vi "orbits_seed_laser_controller.vi"() -> ()   [LabVIEW 2014]
uses:
  <vilib>/Instr/_visa.llb/VISA Configure Serial Port (Instr).vi
panel:
  out "Temp (C)":dbl=35.4
  in  "DISABLE":bool
  in  "ENABLE":bool
  in  "Read":bool
  out "Power (mW)":dbl
  out "Temp (C)":dbl(slide)=35.4 scale=0.0..50.0
  in  "Ethernal COM Port":refnum<visa-resource-name>="COM4"
  in  "Controller Stop":bool
  in  "Control Rate (ms)":u32=1000
  out "Hardware Enabled":bool=TRUE
  out "Software Enabled":bool=TRUE
  out "Temp Stable":bool=TRUE
  in  "Which Temp?":enum16{"ETH", "PUMP", "PCB", "AMP", "CASE"}(ring)
  out "TEC Setpoint":dbl=35.52 format="%#_13g"
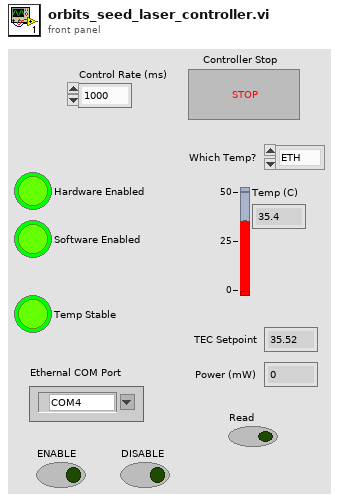
[diagram p1: front panel]
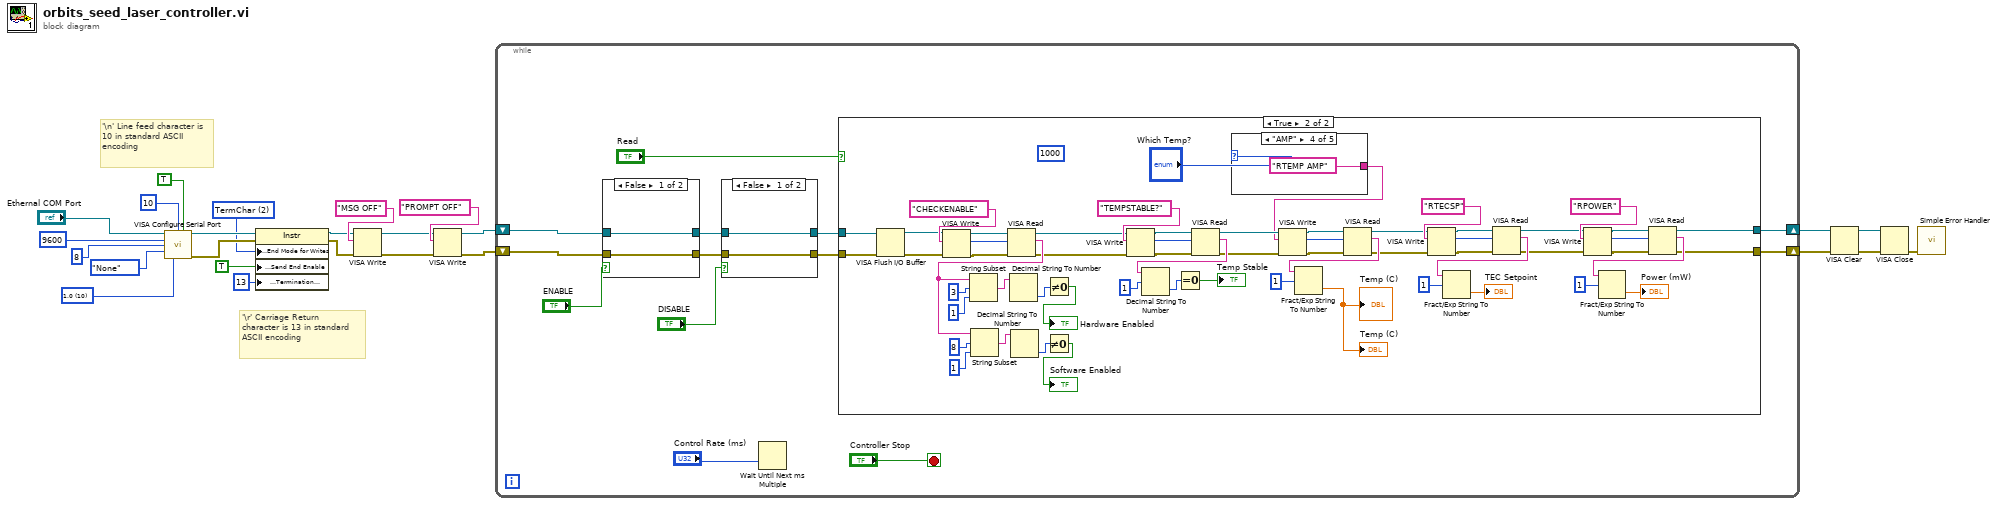
[diagram p0: block diagram]
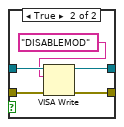
[diagram p2: hidden frame]
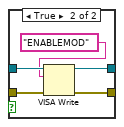
[diagram p3: hidden frame]
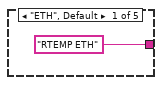
[diagram p5: hidden frame]
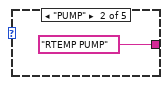
[diagram p6: hidden frame]
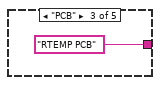
[diagram p7: hidden frame]
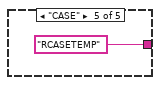
[diagram p8: hidden frame]
diagram:
  w7 = u16 10 items=["1.0"=10, "1.5"=15, "2.0"=20] ("stop bits (10: 1 bit)")
  w21 = u16 2 items=["None", "LastBit", "TermChar", "Break"] ("Serial Settings:Serial End Mode for Writes")
  # "'\\r' Carriage Return character is 13 in standard ASCII encoding"
  # "'\\n' Line feed character is 10 in standard ASCII encoding"
  n1 = call-poly "VISA Configure Serial Port"("VISA resource name"="Ethernal COM Port", "termination char\n(0xA = '\\n' = LF)"=u8 10, "Enable Termination\nChar (T)"=TRUE, "baud rate (9600)"=u32 9600, "data bits (8)"=u16 8, "parity (0:none)"=enum16{"None", "Odd", "Even", "Mark", "Space"}."None", "stop bits (10: 1 bit)"=w7) -> ("VISA resource name out"=w23:refnum<visa-resource-name>, "error out"=w24:errorcluster)  [unwired: 3 in, 4 out]
  n2 = property class="Instr"(reference=w23, error in=w24, "Serial Settings:End Mode for Writes"=w21, "Message Based Settings:Send End Enable"=TRUE, "Message Based Settings:Termination Character"=13) -> (reference out=w12:refnum<visa-resource-name>, error out=w13:errorcluster)
  n3 = VISA Write(VISA resource name=w12, write buffer="MSG OFF" ("Enable 2"), error in (no error)=w13) -> (VISA resource name out=w10:refnum<visa-resource-name>, error out=w9:errorcluster)  [unwired: 1 out]
  n4 = VISA Write(VISA resource name=w10, write buffer="PROMPT OFF" ("Enable 2"), error in (no error)=w9) -> (VISA resource name out=w6:refnum<visa-resource-name>, error out=w5:errorcluster)  [unwired: 1 out]
  n5 = while {
    shift-right: [w35] -> w3
    shift-left: w5 -> [w28]
    shift-right: [w36] -> w4
    shift-left: w6 -> [w29]
    stop <- "Controller Stop" stop-if-true
    n6 = case shown="False" "ENABLE" {
      tunnel: w29 -> [w47 w52]
      tunnel: w28 -> [w46 w51]
      tunnel: [w47 w50] -> w30
      tunnel: [w46 w49] -> w31
      frame False {
      }
      frame True {
        n7 = VISA Write(VISA resource name=w52, write buffer="ENABLEMOD" ("Enable 2"), error in (no error)=w51) -> (VISA resource name out=w50:refnum<visa-resource-name>, error out=w49:errorcluster)  [unwired: 1 out]
      }
    }
    n8 = case shown="False" "DISABLE" {
      tunnel: w30 -> [w40 w45]
      tunnel: w31 -> [w39 w44]
      tunnel: [w40 w43] -> w27
      tunnel: [w39 w42] -> w26
      frame False {
      }
      frame True {
        n9 = VISA Write(VISA resource name=w45, write buffer="DISABLEMOD" ("Enable 2"), error in (no error)=w44) -> (VISA resource name out=w43:refnum<visa-resource-name>, error out=w42:errorcluster)  [unwired: 1 out]
      }
    }
    n10 = Wait Until Next ms Multiple(millisecond multiple="Control Rate (ms)") -> ()  [unwired: 1 out]
    n11 = case shown="True" "Read" {
      tunnel: [w54 w60] -> w36
      tunnel: [w53 w59] -> w35
      tunnel: w27 -> [w54 w58]
      tunnel: w26 -> [w53 w56]
      frame False {
      }
      frame True {
        (unwired) u32 1000 ("Read Count 3")
        n12 = VISA Flush I/O Buffer(VISA resource name=w58, error in (no error)=w56) -> (VISA resource name out=w57:refnum<visa-resource-name>, error out=w55:errorcluster)  [unwired: 1 in]
        n13 = VISA Write(VISA resource name=w57, write buffer="CHECKENABLE" ("Enable 2"), error in (no error)=w55) -> (VISA resource name out=w112:refnum<visa-resource-name>, return count=w65:u32, error out=w111:errorcluster)
        n14 = VISA Read(VISA resource name=w112, byte count=w65, error in (no error)=w111) -> (VISA resource name out=w95:refnum<visa-resource-name>, read buffer=w106:string, error out=w94:errorcluster)  [unwired: 1 out]
        n15 = String Subset(string=w106, offset (0)=3, length (rest)=1) -> (substring=w105:string)
        n16 = String Subset(string=w106, offset (0)=8, length (rest)=1) -> (substring=w104:string)
        n17 = Decimal String To Number(string=w105) -> (number=w103:i32)  [unwired: 2 in, 1 out]
        n18 = Decimal String To Number(string=w104) -> (number=w100:i32)  [unwired: 2 in, 1 out]
        n19 = Not Equal To 0?(x=w100) -> (x != 0?=→"Software Enabled":bool)
        n20 = Not Equal To 0?(x=w103) -> (x != 0?=→"Hardware Enabled":bool)
        n21 = VISA Write(VISA resource name=w95, write buffer="TEMPSTABLE?" ("Enable 2"), error in (no error)=w94) -> (VISA resource name out=w98:refnum<visa-resource-name>, return count=w64:u32, error out=w97:errorcluster)
        n22 = VISA Read(VISA resource name=w98, byte count=w64, error in (no error)=w97) -> (VISA resource name out=w88:refnum<visa-resource-name>, read buffer=w96:string, error out=w87:errorcluster)  [unwired: 1 out]
        n23 = Decimal String To Number(string=w96, offset=1) -> (number=w92:i32)  [unwired: 1 in, 1 out]
        n24 = Equal To 0?(x=w92) -> (x = 0?=→"Temp Stable":bool)
        n25 = case shown="\"AMP\"" "Which Temp?" {
          tunnel: ["RTEMP ETH" ("Enable 2") "RTEMP PUMP" ("Enable 2") "RTEMP PCB" ("Enable 2") "RTEMP AMP" ("Enable 2") "RCASETEMP" ("Enable 2")] -> w86
          frame "ETH", Default {
          }
          frame "PUMP" {
          }
          frame "PCB" {
          }
          frame "AMP" {
          }
          frame "CASE" {
          }
        }
        n26 = VISA Write(VISA resource name=w88, write buffer=w86, error in (no error)=w87) -> (VISA resource name out=w90:refnum<visa-resource-name>, return count=w61:u32, error out=w89:errorcluster)
        n27 = VISA Read(VISA resource name=w90, byte count=w61, error in (no error)=w89) -> (VISA resource name out=w70:refnum<visa-resource-name>, read buffer=w85:string, error out=w69:errorcluster)  [unwired: 1 out]
        n28 = Fract/Exp String To Number(string=w85, offset=1) -> (number=→"Temp (C)" →"Temp (C)":dbl)  [unwired: 2 in, 1 out]
        n29 = VISA Write(VISA resource name=w70, write buffer="RTECSP" ("Enable 2"), error in (no error)=w69) -> (VISA resource name out=w75:refnum<visa-resource-name>, return count=w62:u32, error out=w74:errorcluster)
        n30 = VISA Read(VISA resource name=w75, byte count=w62, error in (no error)=w74) -> (VISA resource name out=w68:refnum<visa-resource-name>, read buffer=w71:string, error out=w67:errorcluster)  [unwired: 1 out]
        n31 = Fract/Exp String To Number(string=w71, offset=1) -> (number=→"TEC Setpoint":dbl)  [unwired: 2 in, 1 out]
        n32 = VISA Write(VISA resource name=w68, write buffer="RPOWER" ("Enable 2"), error in (no error)=w67) -> (VISA resource name out=w83:refnum<visa-resource-name>, return count=w63:u32, error out=w82:errorcluster)
        n33 = VISA Read(VISA resource name=w83, byte count=w63, error in (no error)=w82) -> (VISA resource name out=w60:refnum<visa-resource-name>, read buffer=w77:string, error out=w59:errorcluster)  [unwired: 1 out]
        n34 = Fract/Exp String To Number(string=w77, offset=1) -> (number=→"Power (mW)":dbl)  [unwired: 2 in, 1 out]
      }
    }
  }
  n35 = VISA Clear(VISA resource name=w4, error in (no error)=w3) -> (VISA resource name out=w1:refnum<visa-resource-name>, error out=w2:errorcluster)
  n36 = VISA Close(VISA resource name=w1, error in (no error)=w2) -> (error out=w25:errorcluster)
  n37 = call <vilib>:"Simple Error Handler.vi"("error in (no error)"=w25) -> ()  [unwired: 4 in, 5 out]
